vi "Field vs  IV and Ic distribution_V1.vi"() -> ()   [LabVIEW 2018]
uses:
  <vilib>/LabVIEW Targets/FPGA/cRIO/shared/nicrio_ModuleControls/nicrio_cRIO-9775_RecordDataRates4ChansRing.ctl
  <vilib>/Utility/file.llb/Write Delimited Spreadsheet (DBL).vi
  global.vi
  <resource>/objmgr/ni.dex.rc
  <vilib>/Analysis/NI_AALBase.lvlib
panel:
  in  "Tab Control":enum32{"Field", "cRIO"}(tab)
  in  "KEITHLEY 2400 GPIB Address":string="22"
  in  "Init Ramp Time s":dbl=10.0
  in  "Step Ramp Time s":dbl=1.0
  in  "Field Radius V":dbl=0.25 format="%#_13g"
  in  "Field step V":dbl=0.005 format="%#_13g"
  in  "Field Origin V":dbl format="%#_13g"
  in  "Ramp up first T":bool=TRUE
  in  "Ramp type":string(combo)="Around origin"
  in  "FIeld Scale factor":dbl=10.0
  in  "AI Channel":u8
  in  "Trigger Slope":enum8{"Positive", "Negative"}(ring)
  in  "Dist Record Samples":u32=10000
  in  "cRIO IP":string="//172.22.11.2"
  in  "Data buffer size":i32=1000
  in  "Voltage Scale factor":dbl=0.0001
  in  "Current Scale factor":dbl=2.0
  in  "IV Record Samples":u32=5000
  in  "Gate wait time us":u32=150
  in  "IV Record Data Rate":T1=200 items=["20.000 MS/s (NI 9775)"=1, "10.00 MS/s (NI 9775)"=2, "6.667 MS/s (NI 9775)"=3, "5.000 MS/s (NI 9775)"=4, "2.500 MS/s (NI 9775)"=8, "1.667 MS/s (NI 9775)"=12, "1.250 MS/s (NI 9775)"=16, "1.000 MS/s (NI 9775)"=20, "833.333 KS/s (NI 9775)"=24, "714.286 KS/s (NI 9775)"=28, "625.000 KS/s (NI 9775)"=32, "555.556 KS/s (NI 9775)"=36, "500.000 KS/s (NI 9775)"=40, "454.545 KS/s (NI 9775)"=44, "416.667 KS/s (NI 9775)"=48, "384.615 KS/s (NI 9775)"=52, "357.143 KS/s (NI 9775)"=56, "333.333 KS/s (NI 9775)"=60, "312.500 KS/s (NI 9775)"=64, "294.118 KS/s (NI 9775)"=68, "277.778 KS/s (NI 9775)"=72, "263.158 KS/s (NI 9775)"=76, "250.000 KS/s (NI 9775)"=80, "238.095 KS/s (NI 9775)"=84, "227.273 KS/s (NI 9775)"=88, "217.391 KS/s (NI 9775)"=92, "208.333 KS/s (NI 9775)"=96, "200.000 KS/s (NI 9775)"=100, "192.308 KS/s (NI 9775)"=104, "185.185 KS/s (NI 9775)"=108, "178.571 KS/s (NI 9775)"=112, "172.414 KS/s (NI 9775)"=116, "166.667 KS/s (NI 9775)"=120, "161.290 KS/s (NI 9775)"=124, "156.250 KS/s (NI 9775)"=128, "151.515 KS/s (NI 9775)"=132, "147.059 KS/s (NI 9775)"=136, "142.857 KS/s (NI 9775)"=140, "138.889 KS/s (NI 9775)"=144, "135.135 KS/s (NI 9775)"=148, "131.579 KS/s (NI 9775)"=152, "128.205 KS/s (NI 9775)"=156, "125.000 KS/s (NI 9775)"=160, "121.951 KS/s (NI 9775)"=164, "119.048 KS/s (NI 9775)"=168, "116.279 KS/s (NI 9775)"=172, "113.636 KS/s (NI 9775)"=176, "111.111 KS/s (NI 9775)"=180, "108.696 KS/s (NI 9775)"=184, "106.383 KS/s (NI 9775)"=188, "104.167 KS/s (NI 9775)"=192, "102.041 KS/s (NI 9775)"=196, "100.000 KS/s (NI 9775)"=200, "50.000 KS/s (NI 9775)"=400, "33.333 KS/s (NI 9775)"=600, "25.000 KS/s (NI 9775)"=800, "20.000 KS/s (NI 9775)"=1000, "16.667 KS/s (NI 9775)"=1200, "14.286 KS/s (NI 9775)"=1400, "12.500 KS/s (NI 9775)"=1600, "11.111 KS/s (NI 9775)"=1800, "10.000 KS/s (NI 9775)"=2000, "9.091 KS/s (NI 9775)"=2200, "8.333 KS/s (NI 9775)"=2400, "7.692 KS/s (NI 9775)"=2600, "7.143 KS/s (NI 9775)"=2800, "6.667 KS/s (NI 9775)"=3000, "6.250 KS/s (NI 9775)"=3200, "5.882 KS/s (NI 9775)"=3400, "5.556 KS/s (NI 9775)"=3600, "5.000 KS/s (NI 9775)"=4000, "4.762 KS/s (NI 9775)"=4200, "4.545 KS/s (NI 9775)"=4400, "4.348 KS/s (NI 9775)"=4600, "4.167 KS/s (NI 9775)"=4800, "4.000 KS/s (NI 9775)"=5000, "3.846 KS/s (NI 9775)"=5200, "3.571 KS/s (NI 9775)"=5600, "3.333 KS/s (NI 9775)"=6000, "3.125 KS/s (NI 9775)"=6400, "2.941 KS/s (NI 9775)"=6800, "2.778 KS/s (NI 9775)"=7200, "2.632 KS/s (NI 9775)"=7600, "2.500 KS/s (NI 9775)"=8000, "2.381 KS/s (NI 9775)"=8400, "2.273 KS/s (NI 9775)"=8800, "2.174 KS/s (NI 9775)"=9200, "2.083 KS/s (NI 9775)"=9600, "2.000 KS/s (NI 9775)"=10000, "1.923 KS/s (NI 9775)"=10400, "1.852 KS/s (NI 9775)"=10800, "1.786 KS/s (NI 9775)"=11200, "1.724 KS/s (NI 9775)"=11600, "1.667 KS/s (NI 9775)"=12000, "1.613 KS/s (NI 9775)"=12400, "1.563 KS/s (NI 9775)"=12800, "1.515 KS/s (NI 9775)"=13200, "1.471 KS/s (NI 9775)"=13600, "1.429 KS/s (NI 9775)"=14000, "1.389 KS/s (NI 9775)"=14400, "1.351 KS/s (NI 9775)"=14800, "1.316 KS/s (NI 9775)"=15200, "1.282 KS/s (NI 9775)"=15600, "1.250 KS/s (NI 9775)"=16000, "1.220 KS/s (NI 9775)"=16400, "1.190 KS/s (NI 9775)"=16800, "1.163 KS/s (NI 9775)"=17200, "1.136 KS/s (NI 9775)"=17600, "1.111 KS/s (NI 9775)"=18000, "1.087 KS/s (NI 9775)"=18400, "1.064 KS/s (NI 9775)"=18800, "1.042 KS/s (NI 9775)"=19200, "1.020 KS/s (NI 9775)"=19600, "1.000 KS/s (NI 9775)"=20000, "0.980 KS/s (NI 9775)"=20400, "0.962 KS/s (NI 9775)"=20800, "0.943 KS/s (NI 9775)"=21200, "0.926 KS/s (NI 9775)"=21600, "0.909 KS/s (NI 9775)"=22000, "0.893 KS/s (NI 9775)"=22400, "0.877 KS/s (NI 9775)"=22800, "0.862 KS/s (NI 9775)"=23200, "0.847 KS/s (NI 9775)"=23600, "0.833 KS/s (NI 9775)"=24000, "0.820 KS/s (NI 9775)"=24400, "0.806 KS/s (NI 9775)"=24800, "0.794 KS/s (NI 9775)"=25200, "0.781 KS/s (NI 9775)"=25600, "0.694 KS/s (NI 9775)"=28800, "0.625 KS/s (NI 9775)"=32000, "0.568 KS/s (NI 9775)"=35200, "0.521 KS/s (NI 9775)"=38400, "0.446 KS/s (NI 9775)"=44800, "0.391 KS/s (NI 9775)"=51200, "0.347 KS/s (NI 9775)"=57600, "0.313 KS/s (NI 9775)"=64000]
  in  "Relative threshold":dbl=0.15 format="%#_13g"
  in  "Dist Record Data Rate":T1=1 items=["20.000 MS/s (NI 9775)"=1, "10.00 MS/s (NI 9775)"=2, "6.667 MS/s (NI 9775)"=3, "5.000 MS/s (NI 9775)"=4, "2.500 MS/s (NI 9775)"=8, "1.667 MS/s (NI 9775)"=12, "1.250 MS/s (NI 9775)"=16, "1.000 MS/s (NI 9775)"=20, "833.333 KS/s (NI 9775)"=24, "714.286 KS/s (NI 9775)"=28, "625.000 KS/s (NI 9775)"=32, "555.556 KS/s (NI 9775)"=36, "500.000 KS/s (NI 9775)"=40, "454.545 KS/s (NI 9775)"=44, "416.667 KS/s (NI 9775)"=48, "384.615 KS/s (NI 9775)"=52, "357.143 KS/s (NI 9775)"=56, "333.333 KS/s (NI 9775)"=60, "312.500 KS/s (NI 9775)"=64, "294.118 KS/s (NI 9775)"=68, "277.778 KS/s (NI 9775)"=72, "263.158 KS/s (NI 9775)"=76, "250.000 KS/s (NI 9775)"=80, "238.095 KS/s (NI 9775)"=84, "227.273 KS/s (NI 9775)"=88, "217.391 KS/s (NI 9775)"=92, "208.333 KS/s (NI 9775)"=96, "200.000 KS/s (NI 9775)"=100, "192.308 KS/s (NI 9775)"=104, "185.185 KS/s (NI 9775)"=108, "178.571 KS/s (NI 9775)"=112, "172.414 KS/s (NI 9775)"=116, "166.667 KS/s (NI 9775)"=120, "161.290 KS/s (NI 9775)"=124, "156.250 KS/s (NI 9775)"=128, "151.515 KS/s (NI 9775)"=132, "147.059 KS/s (NI 9775)"=136, "142.857 KS/s (NI 9775)"=140, "138.889 KS/s (NI 9775)"=144, "135.135 KS/s (NI 9775)"=148, "131.579 KS/s (NI 9775)"=152, "128.205 KS/s (NI 9775)"=156, "125.000 KS/s (NI 9775)"=160, "121.951 KS/s (NI 9775)"=164, "119.048 KS/s (NI 9775)"=168, "116.279 KS/s (NI 9775)"=172, "113.636 KS/s (NI 9775)"=176, "111.111 KS/s (NI 9775)"=180, "108.696 KS/s (NI 9775)"=184, "106.383 KS/s (NI 9775)"=188, "104.167 KS/s (NI 9775)"=192, "102.041 KS/s (NI 9775)"=196, "100.000 KS/s (NI 9775)"=200, "50.000 KS/s (NI 9775)"=400, "33.333 KS/s (NI 9775)"=600, "25.000 KS/s (NI 9775)"=800, "20.000 KS/s (NI 9775)"=1000, "16.667 KS/s (NI 9775)"=1200, "14.286 KS/s (NI 9775)"=1400, "12.500 KS/s (NI 9775)"=1600, "11.111 KS/s (NI 9775)"=1800, "10.000 KS/s (NI 9775)"=2000, "9.091 KS/s (NI 9775)"=2200, "8.333 KS/s (NI 9775)"=2400, "7.692 KS/s (NI 9775)"=2600, "7.143 KS/s (NI 9775)"=2800, "6.667 KS/s (NI 9775)"=3000, "6.250 KS/s (NI 9775)"=3200, "5.882 KS/s (NI 9775)"=3400, "5.556 KS/s (NI 9775)"=3600, "5.000 KS/s (NI 9775)"=4000, "4.762 KS/s (NI 9775)"=4200, "4.545 KS/s (NI 9775)"=4400, "4.348 KS/s (NI 9775)"=4600, "4.167 KS/s (NI 9775)"=4800, "4.000 KS/s (NI 9775)"=5000, "3.846 KS/s (NI 9775)"=5200, "3.571 KS/s (NI 9775)"=5600, "3.333 KS/s (NI 9775)"=6000, "3.125 KS/s (NI 9775)"=6400, "2.941 KS/s (NI 9775)"=6800, "2.778 KS/s (NI 9775)"=7200, "2.632 KS/s (NI 9775)"=7600, "2.500 KS/s (NI 9775)"=8000, "2.381 KS/s (NI 9775)"=8400, "2.273 KS/s (NI 9775)"=8800, "2.174 KS/s (NI 9775)"=9200, "2.083 KS/s (NI 9775)"=9600, "2.000 KS/s (NI 9775)"=10000, "1.923 KS/s (NI 9775)"=10400, "1.852 KS/s (NI 9775)"=10800, "1.786 KS/s (NI 9775)"=11200, "1.724 KS/s (NI 9775)"=11600, "1.667 KS/s (NI 9775)"=12000, "1.613 KS/s (NI 9775)"=12400, "1.563 KS/s (NI 9775)"=12800, "1.515 KS/s (NI 9775)"=13200, "1.471 KS/s (NI 9775)"=13600, "1.429 KS/s (NI 9775)"=14000, "1.389 KS/s (NI 9775)"=14400, "1.351 KS/s (NI 9775)"=14800, "1.316 KS/s (NI 9775)"=15200, "1.282 KS/s (NI 9775)"=15600, "1.250 KS/s (NI 9775)"=16000, "1.220 KS/s (NI 9775)"=16400, "1.190 KS/s (NI 9775)"=16800, "1.163 KS/s (NI 9775)"=17200, "1.136 KS/s (NI 9775)"=17600, "1.111 KS/s (NI 9775)"=18000, "1.087 KS/s (NI 9775)"=18400, "1.064 KS/s (NI 9775)"=18800, "1.042 KS/s (NI 9775)"=19200, "1.020 KS/s (NI 9775)"=19600, "1.000 KS/s (NI 9775)"=20000, "0.980 KS/s (NI 9775)"=20400, "0.962 KS/s (NI 9775)"=20800, "0.943 KS/s (NI 9775)"=21200, "0.926 KS/s (NI 9775)"=21600, "0.909 KS/s (NI 9775)"=22000, "0.893 KS/s (NI 9775)"=22400, "0.877 KS/s (NI 9775)"=22800, "0.862 KS/s (NI 9775)"=23200, "0.847 KS/s (NI 9775)"=23600, "0.833 KS/s (NI 9775)"=24000, "0.820 KS/s (NI 9775)"=24400, "0.806 KS/s (NI 9775)"=24800, "0.794 KS/s (NI 9775)"=25200, "0.781 KS/s (NI 9775)"=25600, "0.694 KS/s (NI 9775)"=28800, "0.625 KS/s (NI 9775)"=32000, "0.568 KS/s (NI 9775)"=35200, "0.521 KS/s (NI 9775)"=38400, "0.446 KS/s (NI 9775)"=44800, "0.391 KS/s (NI 9775)"=51200, "0.347 KS/s (NI 9775)"=57600, "0.313 KS/s (NI 9775)"=64000]
  in  "Zero avg":i32=500
  out "Threshold":dbl=0.1399287109375
  in  "Stop loop":bool
  out "Current Field mT":dbl=-0.050000000000000044
  out "Current Field V":dbl=-0.0050000000000000044
  in  "Name":string="book379"
  in  "Contour plot folder":path=path "C:/Users/gyue/Box Sync/Guang Yue/data/Contour plot"
  out "Histogram Graph":T2(graph)={"X Values"=[9.09032470703125, 9.09519287109375, 9.100061035156251, 9.104929199218752, 9.109797363281253, 9.114665527343753, 9.119533691406254, 9.124401855468754, 9.129270019531255, 9.134138183593755, 9.139006347656256, 9.143874511718757, 9.148742675781257, 9.153610839843758, 9.158479003906258, 9.163347167968759, 9.16821533203126, 9.17308349609376, 9.17795166015626, 9.182819824218761, 9.187687988281262, 9.192556152343762, 9.197424316406263, 9.202292480468763, 9.207160644531264, 9.212028808593764, 9.216896972656265, 9.221765136718766, 9.226633300781266, 9.231501464843767, 9.236369628906267, 9.241237792968768, 9.246105957031268, 9.250974121093769, 9.25584228515627, 9.26071044921877, 9.26557861328127, 9.270446777343771, 9.275314941406272, 9.280183105468772, 9.285051269531273, 9.289919433593774, 9.294787597656274, 9.299655761718775, 9.304523925781275, 9.309392089843776, 9.314260253906276, 9.319128417968777, 9.323996582031278, 9.328864746093778, 9.333732910156279, 9.33860107421878, 9.34346923828128, 9.34833740234378, 9.353205566406281, 9.358073730468782, 9.362941894531282, 9.367810058593783, 9.372678222656283, 9.377546386718784, 9.382414550781284, 9.387282714843785, 9.392150878906286, 9.397019042968786, 9.401887207031287, 9.406755371093787, 9.411623535156288, 9.416491699218788, 9.421359863281289, 9.42622802734379, 9.43109619140629, 9.43596435546879, 9.440832519531291, 9.445700683593792, 9.450568847656292, 9.455437011718793, 9.460305175781293, 9.465173339843794, 9.470041503906295, 9.474909667968795, 9.479777832031296, 9.484645996093796, 9.489514160156297, 9.494382324218797, 9.499250488281298, 9.504118652343799, 9.5089868164063, 9.5138549804688, 9.5187231445313, 9.5235913085938, 9.528459472656301, 9.533327636718802, 9.538195800781303, 9.543063964843803, 9.547932128906304, 9.552800292968804, 9.557668457031305, 9.562536621093805, 9.567404785156306, 9.572272949218807], "Histogram: h(x)"=[1, 0, 0, 1, 1, 1, 0, 5, 0, 4, 3, 0, 0, 5, 6, 15, 9, 18, 14, 21, 6, 18, 23, 34, 38, 22, 54, 57, 74, 39, 98, 103, 123, 63, 111, 190, 161, 108, 207, 263, 218, 147, 272, 308, 339, 142, 370, 304, 377, 152, 388, 375, 351, 359, 135, 364, 278, 319, 146, 320, 254, 252, 130, 192, 217, 177, 103, 150, 140, 114, 62, 113, 105, 82, 24, 58, 42, 47, 16, 34, 33, 19, 18, 4, 13, 9, 7, 3, 5, 4, 2, 1, 2, 1, 2, 2, 1, 0, 0, 2]}
  out "Ic parameters":T3={"Records Num"=10000, "AI Trigger Configuration"={"Trigger Slope"=enum."Positive", "Trigger Level"=0.139892578125, "Hystesis Value"=0.1328125, "AI Channel"=0}, "Record PreTrigger Samples"=1, "Record Samples"=16, "Ic Cut off or curve"=TRUE, "Gate wait time us"=150, "Record Data Rate"=1} {"Record Data Rate" items=["20.000 MS/s (NI 9775)"=1, "10.00 MS/s (NI 9775)"=2, "6.667 MS/s (NI 9775)"=3, "5.000 MS/s (NI 9775)"=4, "2.500 MS/s (NI 9775)"=8, "1.667 MS/s (NI 9775)"=12, "1.250 MS/s (NI 9775)"=16, "1.000 MS/s (NI 9775)"=20, "833.333 KS/s (NI 9775)"=24, "714.286 KS/s (NI 9775)"=28, "625.000 KS/s (NI 9775)"=32, "555.556 KS/s (NI 9775)"=36, "500.000 KS/s (NI 9775)"=40, "454.545 KS/s (NI 9775)"=44, "416.667 KS/s (NI 9775)"=48, "384.615 KS/s (NI 9775)"=52, "357.143 KS/s (NI 9775)"=56, "333.333 KS/s (NI 9775)"=60, "312.500 KS/s (NI 9775)"=64, "294.118 KS/s (NI 9775)"=68, "277.778 KS/s (NI 9775)"=72, "263.158 KS/s (NI 9775)"=76, "250.000 KS/s (NI 9775)"=80, "238.095 KS/s (NI 9775)"=84, "227.273 KS/s (NI 9775)"=88, "217.391 KS/s (NI 9775)"=92, "208.333 KS/s (NI 9775)"=96, "200.000 KS/s (NI 9775)"=100, "192.308 KS/s (NI 9775)"=104, "185.185 KS/s (NI 9775)"=108, "178.571 KS/s (NI 9775)"=112, "172.414 KS/s (NI 9775)"=116, "166.667 KS/s (NI 9775)"=120, "161.290 KS/s (NI 9775)"=124, "156.250 KS/s (NI 9775)"=128, "151.515 KS/s (NI 9775)"=132, "147.059 KS/s (NI 9775)"=136, "142.857 KS/s (NI 9775)"=140, "138.889 KS/s (NI 9775)"=144, "135.135 KS/s (NI 9775)"=148, "131.579 KS/s (NI 9775)"=152, "128.205 KS/s (NI 9775)"=156, "125.000 KS/s (NI 9775)"=160, "121.951 KS/s (NI 9775)"=164, "119.048 KS/s (NI 9775)"=168, "116.279 KS/s (NI 9775)"=172, "113.636 KS/s (NI 9775)"=176, "111.111 KS/s (NI 9775)"=180, "108.696 KS/s (NI 9775)"=184, "106.383 KS/s (NI 9775)"=188, "104.167 KS/s (NI 9775)"=192, "102.041 KS/s (NI 9775)"=196, "100.000 KS/s (NI 9775)"=200, "50.000 KS/s (NI 9775)"=400, "33.333 KS/s (NI 9775)"=600, "25.000 KS/s (NI 9775)"=800, "20.000 KS/s (NI 9775)"=1000, "16.667 KS/s (NI 9775)"=1200, "14.286 KS/s (NI 9775)"=1400, "12.500 KS/s (NI 9775)"=1600, "11.111 KS/s (NI 9775)"=1800, "10.000 KS/s (NI 9775)"=2000, "9.091 KS/s (NI 9775)"=2200, "8.333 KS/s (NI 9775)"=2400, "7.692 KS/s (NI 9775)"=2600, "7.143 KS/s (NI 9775)"=2800, "6.667 KS/s (NI 9775)"=3000, "6.250 KS/s (NI 9775)"=3200, "5.882 KS/s (NI 9775)"=3400, "5.556 KS/s (NI 9775)"=3600, "5.000 KS/s (NI 9775)"=4000, "4.762 KS/s (NI 9775)"=4200, "4.545 KS/s (NI 9775)"=4400, "4.348 KS/s (NI 9775)"=4600, "4.167 KS/s (NI 9775)"=4800, "4.000 KS/s (NI 9775)"=5000, "3.846 KS/s (NI 9775)"=5200, "3.571 KS/s (NI 9775)"=5600, "3.333 KS/s (NI 9775)"=6000, "3.125 KS/s (NI 9775)"=6400, "2.941 KS/s (NI 9775)"=6800, "2.778 KS/s (NI 9775)"=7200, "2.632 KS/s (NI 9775)"=7600, "2.500 KS/s (NI 9775)"=8000, "2.381 KS/s (NI 9775)"=8400, "2.273 KS/s (NI 9775)"=8800, "2.174 KS/s (NI 9775)"=9200, "2.083 KS/s (NI 9775)"=9600, "2.000 KS/s (NI 9775)"=10000, "1.923 KS/s (NI 9775)"=10400, "1.852 KS/s (NI 9775)"=10800, "1.786 KS/s (NI 9775)"=11200, "1.724 KS/s (NI 9775)"=11600, "1.667 KS/s (NI 9775)"=12000, "1.613 KS/s (NI 9775)"=12400, "1.563 KS/s (NI 9775)"=12800, "1.515 KS/s (NI 9775)"=13200, "1.471 KS/s (NI 9775)"=13600, "1.429 KS/s (NI 9775)"=14000, "1.389 KS/s (NI 9775)"=14400, "1.351 KS/s (NI 9775)"=14800, "1.316 KS/s (NI 9775)"=15200, "1.282 KS/s (NI 9775)"=15600, "1.250 KS/s (NI 9775)"=16000, "1.220 KS/s (NI 9775)"=16400, "1.190 KS/s (NI 9775)"=16800, "1.163 KS/s (NI 9775)"=17200, "1.136 KS/s (NI 9775)"=17600, "1.111 KS/s (NI 9775)"=18000, "1.087 KS/s (NI 9775)"=18400, "1.064 KS/s (NI 9775)"=18800, "1.042 KS/s (NI 9775)"=19200, "1.020 KS/s (NI 9775)"=19600, "1.000 KS/s (NI 9775)"=20000, "0.980 KS/s (NI 9775)"=20400, "0.962 KS/s (NI 9775)"=20800, "0.943 KS/s (NI 9775)"=21200, "0.926 KS/s (NI 9775)"=21600, "0.909 KS/s (NI 9775)"=22000, "0.893 KS/s (NI 9775)"=22400, "0.877 KS/s (NI 9775)"=22800, "0.862 KS/s (NI 9775)"=23200, "0.847 KS/s (NI 9775)"=23600, "0.833 KS/s (NI 9775)"=24000, "0.820 KS/s (NI 9775)"=24400, "0.806 KS/s (NI 9775)"=24800, "0.794 KS/s (NI 9775)"=25200, "0.781 KS/s (NI 9775)"=25600, "0.694 KS/s (NI 9775)"=28800, "0.625 KS/s (NI 9775)"=32000, "0.568 KS/s (NI 9775)"=35200, "0.521 KS/s (NI 9775)"=38400, "0.446 KS/s (NI 9775)"=44800, "0.391 KS/s (NI 9775)"=51200, "0.347 KS/s (NI 9775)"=57600, "0.313 KS/s (NI 9775)"=64000]}
  out "IV parameters":T3={"Records Num"=1, "AI Trigger Configuration"={"Trigger Slope"=enum."Positive", "Trigger Level"=0.10009765625, "Hystesis Value"=0.094970703125, "AI Channel"=0}, "Record PreTrigger Samples"=1, "Record Samples"=5000, "Ic Cut off or curve"=FALSE, "Gate wait time us"=150, "Record Data Rate"=200} {"Record Data Rate" items=["20.000 MS/s (NI 9775)"=1, "10.00 MS/s (NI 9775)"=2, "6.667 MS/s (NI 9775)"=3, "5.000 MS/s (NI 9775)"=4, "2.500 MS/s (NI 9775)"=8, "1.667 MS/s (NI 9775)"=12, "1.250 MS/s (NI 9775)"=16, "1.000 MS/s (NI 9775)"=20, "833.333 KS/s (NI 9775)"=24, "714.286 KS/s (NI 9775)"=28, "625.000 KS/s (NI 9775)"=32, "555.556 KS/s (NI 9775)"=36, "500.000 KS/s (NI 9775)"=40, "454.545 KS/s (NI 9775)"=44, "416.667 KS/s (NI 9775)"=48, "384.615 KS/s (NI 9775)"=52, "357.143 KS/s (NI 9775)"=56, "333.333 KS/s (NI 9775)"=60, "312.500 KS/s (NI 9775)"=64, "294.118 KS/s (NI 9775)"=68, "277.778 KS/s (NI 9775)"=72, "263.158 KS/s (NI 9775)"=76, "250.000 KS/s (NI 9775)"=80, "238.095 KS/s (NI 9775)"=84, "227.273 KS/s (NI 9775)"=88, "217.391 KS/s (NI 9775)"=92, "208.333 KS/s (NI 9775)"=96, "200.000 KS/s (NI 9775)"=100, "192.308 KS/s (NI 9775)"=104, "185.185 KS/s (NI 9775)"=108, "178.571 KS/s (NI 9775)"=112, "172.414 KS/s (NI 9775)"=116, "166.667 KS/s (NI 9775)"=120, "161.290 KS/s (NI 9775)"=124, "156.250 KS/s (NI 9775)"=128, "151.515 KS/s (NI 9775)"=132, "147.059 KS/s (NI 9775)"=136, "142.857 KS/s (NI 9775)"=140, "138.889 KS/s (NI 9775)"=144, "135.135 KS/s (NI 9775)"=148, "131.579 KS/s (NI 9775)"=152, "128.205 KS/s (NI 9775)"=156, "125.000 KS/s (NI 9775)"=160, "121.951 KS/s (NI 9775)"=164, "119.048 KS/s (NI 9775)"=168, "116.279 KS/s (NI 9775)"=172, "113.636 KS/s (NI 9775)"=176, "111.111 KS/s (NI 9775)"=180, "108.696 KS/s (NI 9775)"=184, "106.383 KS/s (NI 9775)"=188, "104.167 KS/s (NI 9775)"=192, "102.041 KS/s (NI 9775)"=196, "100.000 KS/s (NI 9775)"=200, "50.000 KS/s (NI 9775)"=400, "33.333 KS/s (NI 9775)"=600, "25.000 KS/s (NI 9775)"=800, "20.000 KS/s (NI 9775)"=1000, "16.667 KS/s (NI 9775)"=1200, "14.286 KS/s (NI 9775)"=1400, "12.500 KS/s (NI 9775)"=1600, "11.111 KS/s (NI 9775)"=1800, "10.000 KS/s (NI 9775)"=2000, "9.091 KS/s (NI 9775)"=2200, "8.333 KS/s (NI 9775)"=2400, "7.692 KS/s (NI 9775)"=2600, "7.143 KS/s (NI 9775)"=2800, "6.667 KS/s (NI 9775)"=3000, "6.250 KS/s (NI 9775)"=3200, "5.882 KS/s (NI 9775)"=3400, "5.556 KS/s (NI 9775)"=3600, "5.000 KS/s (NI 9775)"=4000, "4.762 KS/s (NI 9775)"=4200, "4.545 KS/s (NI 9775)"=4400, "4.348 KS/s (NI 9775)"=4600, "4.167 KS/s (NI 9775)"=4800, "4.000 KS/s (NI 9775)"=5000, "3.846 KS/s (NI 9775)"=5200, "3.571 KS/s (NI 9775)"=5600, "3.333 KS/s (NI 9775)"=6000, "3.125 KS/s (NI 9775)"=6400, "2.941 KS/s (NI 9775)"=6800, "2.778 KS/s (NI 9775)"=7200, "2.632 KS/s (NI 9775)"=7600, "2.500 KS/s (NI 9775)"=8000, "2.381 KS/s (NI 9775)"=8400, "2.273 KS/s (NI 9775)"=8800, "2.174 KS/s (NI 9775)"=9200, "2.083 KS/s (NI 9775)"=9600, "2.000 KS/s (NI 9775)"=10000, "1.923 KS/s (NI 9775)"=10400, "1.852 KS/s (NI 9775)"=10800, "1.786 KS/s (NI 9775)"=11200, "1.724 KS/s (NI 9775)"=11600, "1.667 KS/s (NI 9775)"=12000, "1.613 KS/s (NI 9775)"=12400, "1.563 KS/s (NI 9775)"=12800, "1.515 KS/s (NI 9775)"=13200, "1.471 KS/s (NI 9775)"=13600, "1.429 KS/s (NI 9775)"=14000, "1.389 KS/s (NI 9775)"=14400, "1.351 KS/s (NI 9775)"=14800, "1.316 KS/s (NI 9775)"=15200, "1.282 KS/s (NI 9775)"=15600, "1.250 KS/s (NI 9775)"=16000, "1.220 KS/s (NI 9775)"=16400, "1.190 KS/s (NI 9775)"=16800, "1.163 KS/s (NI 9775)"=17200, "1.136 KS/s (NI 9775)"=17600, "1.111 KS/s (NI 9775)"=18000, "1.087 KS/s (NI 9775)"=18400, "1.064 KS/s (NI 9775)"=18800, "1.042 KS/s (NI 9775)"=19200, "1.020 KS/s (NI 9775)"=19600, "1.000 KS/s (NI 9775)"=20000, "0.980 KS/s (NI 9775)"=20400, "0.962 KS/s (NI 9775)"=20800, "0.943 KS/s (NI 9775)"=21200, "0.926 KS/s (NI 9775)"=21600, "0.909 KS/s (NI 9775)"=22000, "0.893 KS/s (NI 9775)"=22400, "0.877 KS/s (NI 9775)"=22800, "0.862 KS/s (NI 9775)"=23200, "0.847 KS/s (NI 9775)"=23600, "0.833 KS/s (NI 9775)"=24000, "0.820 KS/s (NI 9775)"=24400, "0.806 KS/s (NI 9775)"=24800, "0.794 KS/s (NI 9775)"=25200, "0.781 KS/s (NI 9775)"=25600, "0.694 KS/s (NI 9775)"=28800, "0.625 KS/s (NI 9775)"=32000, "0.568 KS/s (NI 9775)"=35200, "0.521 KS/s (NI 9775)"=38400, "0.446 KS/s (NI 9775)"=44800, "0.391 KS/s (NI 9775)"=51200, "0.347 KS/s (NI 9775)"=57600, "0.313 KS/s (NI 9775)"=64000]}
  out "XY Graph":cluster{"Y":dbl[], "Y":dbl[]}[](graph)
  in  "stop":bool
  out "error out":errorcluster={"status"=FALSE, "code"=180121605, "source"="Shared Variable in Field vs  IV and Ic distribution.vi<APPEND>\nThis error or warning occurred while writing the following Shared Variable:\n\\\\NI-cRIO-9063-01bc8cc6\\network varibles\\RT Stop\n\\\\172.22.11.2\\network varibles\\RT Stop"}
  # "Voltage x factor=mT"
  # "Distribution setting"
  # "IV setting"
  # "Voltage x factor=uA"
  # "Voltage x factor=V"
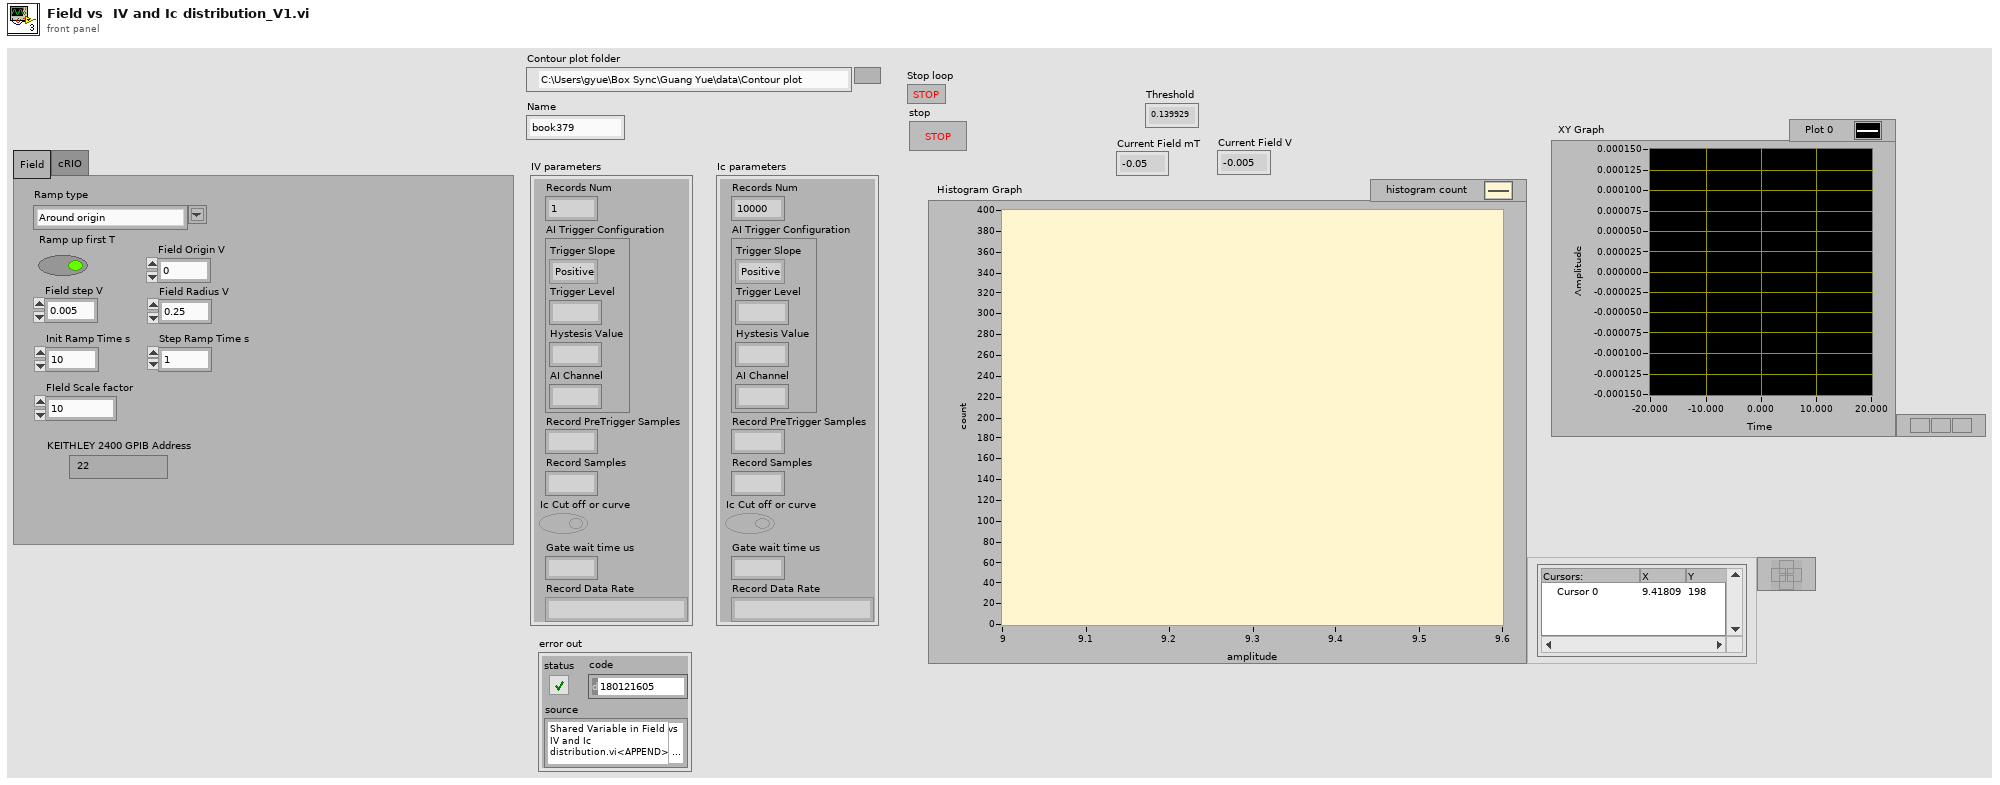
[diagram p1: front panel]
types:
  T1 = typedef "nicrio_cRIO-9775_RecordDataRates4ChansRing.ctl" = u16
  T2 = cluster{"X Values":dbl[], "Histogram: h(x)":i32[]}
  T3 = cluster{"Records Num":i32, "AI Trigger Configuration":cluster{"Trigger Slope":enum8{"Positive", "Negative"}, "Trigger Level":fxp<+/-,17,5>, "Hystesis Value":fxp<+,16,4>, "AI Channel":u8}, "Record PreTrigger Samples":u32, "Record Samples":u32, "Ic Cut off or curve":bool, "Gate wait time us":u32, "Record Data Rate":T1}
  T4 = cluster{"Trigger Slope":enum8{"Positive", "Negative"}, "Trigger Level":fxp<+/-,17,5>, "Hystesis Value":fxp<+,16,4>, "AI Channel":u8}
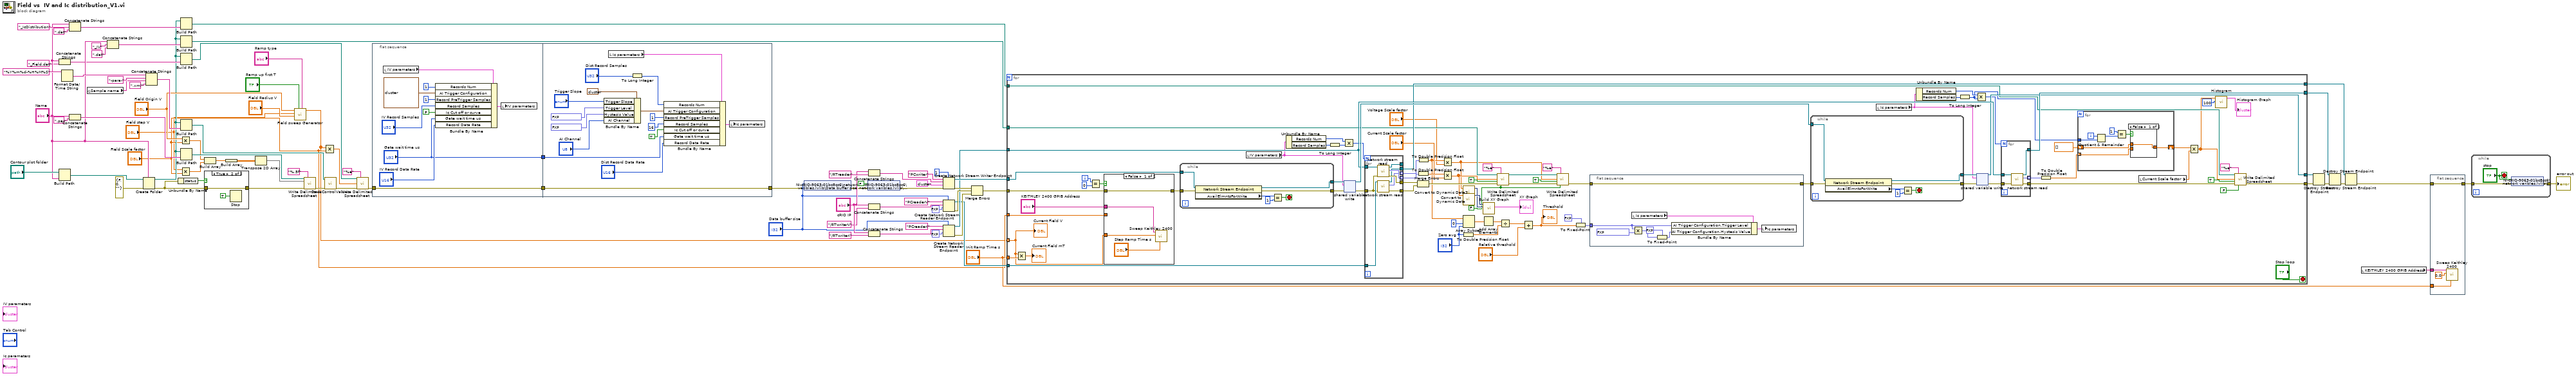
[diagram p0: block diagram]
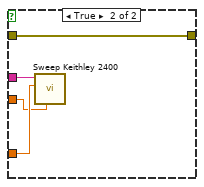
[diagram p3: hidden frame]
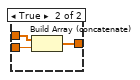
[diagram p4: hidden frame]
diagram:
  n1 = Concatenate Strings("Name", "_Field.dat" ("string")) -> (w14:string)
  n2 = Build Path(base path="Contour plot folder", name or relative path="Name") -> (appended path=w40:path)
  n3 = Format Date/Time String(time format string (%c)="%Y%m%d-%H%M%S") -> (date/time string=w35:string)  [unwired: 2 in]
  n4 = Concatenate Strings("Name", "_IcDistribution" ("string"), ".dat" ("string")) -> (w26:string)
  n5 = Concatenate Strings("Name", ".par" ("string")) -> (w47:string)
  n6 = global read "global.vi" "Sample name"() -> (w34:string)
  n7 = Concatenate Strings("Name", "_IV" ("string"), ".dat" ("string")) -> (w41:string)
  n8 = Create Folder(prompt (Create Folder)="Name", path (use dialog)=w40, error in=errorcluster {"status"=FALSE, "code"=0, "source"=""}) -> (created path=w13:path, error out=w37:errorcluster)  [unwired: 1 out]
  n9 = Concatenate Strings(w35, "-para-" ("string"), w34, ".xml" ("string")) -> (w51:string)
  n10 = Unbundle By Name(w37) -> ("status"=w38:bool)
  n11 = Multiply(x="Field Origin V", y="FIeld Scale factor") -> (x*y=w33:dbl)
  n12 = Multiply(x="Field step V", y="FIeld Scale factor") -> (x*y=w32:dbl)
  n13 = Build Path(base path=w13, name or relative path=w26) -> (appended path=w24:path)
  n14 = Build Path(base path=w13, name or relative path=w41) -> (appended path=w25:path)
  n15 = Build Path(base path=w13, name or relative path=w14) -> (appended path=w12:path)
  n16 = Build Path(base path=w13, name or relative path=w51) -> (appended path=w49:path)
  n17 = Build Path(base path=w13, name or relative path=w47) -> (appended path=w46:path)
  n18 = Build Array(w33, w32) -> (w44:dbl[])
  n19 = case shown="True" w38 {
    tunnel: [w87 w89] -> w36
    tunnel: w37 -> [w87 w89]
    frame False {
    }
    frame True {
      n20 = Stop(stop? (T)=TRUE) -> ()
    }
  }
  n21 = Build Array(w44) -> (w43:dbl[][])
  n22 = Transpose 2D Array(2D array=w43) -> (transposed array=w42:dbl[][])
  n23 = call "Field sweep Generator.vi"("Ramp type"="Ramp type", "Ramp up first T"="Ramp up first T", "Field Radius V"="Field Radius V", "Field step V"="Field step V", "Field Origin V"="Field Origin V") -> ("output array"=w3:dbl[])  [unwired: 6 in]
  n24 = call-poly <vilib>:"Write Delimited Spreadsheet.vi"("file path (dialog if empty)"=w46, "format (%.3f)"="%.5f", "2D data"=w42, "error in (no error)"=w36) -> ("error out"=w39:errorcluster)  [unwired: 10 in, 1 out]
  n25 = Multiply(x=w3, y="FIeld Scale factor") -> (x*y=w9:dbl[])
  n26 = call "SaveControlValues.vi"("XML File Path"=w49, "error in (no error)"=w39) -> ("error out"=w8:errorcluster)  [unwired: 8 in]
  n27 = call-poly <vilib>:"Write Delimited Spreadsheet.vi"("file path (dialog if empty)"=w12, "format (%.3f)"="%e", "1D data"=w9, "error in (no error)"=w8) -> ("error out"=w7:errorcluster)  [unwired: 10 in, 1 out]
  n28 = flat-sequence {
    tunnel: w7 -> [w99]
    tunnel: [w99] -> w5
    tunnel: ["Gate wait time us"] -> w4
    tunnel: [w115] -> w6
    tunnel: w5 -> [w115]
    tunnel: w4 -> [w107]
    frame #0 {
      n29 = local read "IV parameters"() -> (w98:T3)
      n30 = Bundle By Name(cluster=w98, "Records Num"=1, "AI Trigger Configuration"=T4 {"Trigger Slope"=enum."Positive", "Trigger Level"=0.10009765625, "Hystesis Value"=0.094970703125, "AI Channel"=0}, "Record PreTrigger Samples"=u32 1, "Record Samples"="IV Record Samples", "Ic Cut off or curve"=FALSE, "Gate wait time us"="Gate wait time us", "Record Data Rate"="IV Record Data Rate") -> (w90:T3)
      n31 = local write "IV parameters"(w90) -> ()
    }
    frame #1 {
      n32 = Bundle By Name(cluster=T4 {"Trigger Slope"=enum."Positive", "Trigger Level"=0.1708984375, "Hystesis Value"=0.162353515625, "AI Channel"=0} ("AI Trigger Configuration"), "Trigger Slope"="Trigger Slope", "Trigger Level"=fxp<+/-,17,5> 0.14990234375, "Hystesis Value"=fxp<+,16,4> 0.10009765625, "AI Channel"="AI Channel") -> (w103:T4)
      n33 = local read "Ic parameters"() -> (w114:T3)
      n34 = To Long Integer(number="Dist Record Samples") -> (32bit integer=w112:i32)
      n35 = Bundle By Name(cluster=w114, "Records Num"=w112, "AI Trigger Configuration"=w103, "Record PreTrigger Samples"=u32 1, "Record Samples"=u32 16, "Ic Cut off or curve"=TRUE, "Gate wait time us"=w107, "Record Data Rate"="Dist Record Data Rate") -> (w102:T3)
      n36 = local write "Ic parameters"(w102) -> ()
    }
  }
  n37 = shared-variable "NI-cRIO-9063-01bc8cc6\\network varibles.lvlib\\Data buffer size"("Data buffer size", error in=w6) -> (error out=w64:errorcluster)
  n38 = shared-variable "NI-cRIO-9063-01bc8cc6\\network varibles.lvlib\\RT Stop"(FALSE ("RT Stop"), error in=w64) -> (error out=w72:errorcluster)
  n39 = Concatenate Strings("cRIO IP", "/RTreader" ("string")) -> (w82:string)
  n40 = Concatenate Strings("cRIO IP", "/RTwriterV" ("string")) -> (w74:string)
  n41 = Concatenate Strings("cRIO IP", "/RTwriterI" ("string")) -> (w66:string)
  n42 = Create Network Stream Writer Endpoint(7:1 ("writer buffer size"), 8:w72, 9:T3 {"Records Num"=0, "AI Trigger Configuration"={"Trigger Slope"=enum."Positive", "Trigger Level"=0.0, "Hystesis Value"=0.0, "AI Channel"=0}, "Record PreTrigger Samples"=0, "Record Samples"=0, "Ic Cut off or curve"=FALSE, "Gate wait time us"=0, "Record Data Rate"=1} ("Parameters 4"), 10:w82, 11:"PCwriter" ("writer name")) -> (0:w80:errorcluster, 3:w79:refnum<k21>)  [unwired: 2 in]
  n43 = Create Network Stream Reader Endpoint(7:"Data buffer size", 9:fxp<+/-,17,5> 0.0, 10:w74, 11:"PCreaderV" ("reader name")) -> (0:w71:errorcluster, 3:w58:refnum<k21>)  [unwired: 3 in]
  n44 = Create Network Stream Reader Endpoint(7:"Data buffer size", 9:fxp<+/-,17,5> 0.0, 10:w66, 11:"PCreaderI" ("reader name")) -> (0:w63:errorcluster, 3:w61:refnum<k21>)  [unwired: 3 in]
  n45 = Merge Errors(w80, w71, w63) -> (w78:errorcluster)
  n46 = for {
    tunnel: w79 -> [w196]
    tunnel: [w185] -> w59
    tunnel: w78 -> [w158]
    tunnel: [w143] -> w56
    tunnel: w61 -> [w190]
    tunnel: [w188] -> w60
    tunnel: w58 -> [w173]
    tunnel: [w172] -> w57
    tunnel: "FIeld Scale factor" -> [w162]
    tunnel: "Init Ramp Time s" -> [w159]
    tunnel: w25 -> [w149]
    tunnel: w24 -> [w141]
    tunnel: w3 -> [w126] mode=indexing
    i -> [w163]
    stop <- "Stop loop" stop-if-true
    w127 = FALSE ("transpose? (no:F)")
    n47 = Multiply(x=w126, y=w162) -> (x*y=→"Current Field mT":dbl)
    n48 = Equal?(x=w163, y=0) -> (x = y?=w161:bool)
    n49 = case shown="False" w161 {
      tunnel: w158 -> [w209 w210]
      tunnel: [w209 w210] -> w157
      tunnel: w126 -> [w206 w213]
      tunnel: "KEITHLEY 2400 GPIB Address" -> [w207 w212]
      tunnel: w159 -> [_ w211]
      frame False {
        n50 = call "Sweep Keithley 2400.vi"("Ramp Time (s)"="Step Ramp Time s", "final gate voltage (V)"=w206, "KEITHLEY 2400 GPIB Address"=w207) -> ()  [unwired: 7 in, 2 out]
      }
      frame True {
        n51 = call "Sweep Keithley 2400.vi"("Ramp Time (s)"=w211, "final gate voltage (V)"=w213, "KEITHLEY 2400 GPIB Address"=w212) -> ()  [unwired: 7 in, 2 out]
      }
    }
    n52 = while {
      tunnel: w196 -> [w253]
      tunnel: w157 -> [w252]
      tunnel: [w248] -> w197
      tunnel: [w247] -> w195
      stop <- w249 stop-if-true
      n53 = property class="Network Stream Endpoint"(reference=w253, error in=w252) -> (reference out=w248:refnum<k21>, error out=w247:errorcluster, "AvailElmntsForWrite"=w251:i32)
      n54 = Equal?(x=w251, y=1) -> (x = y?=w249:bool)
    }
    n55 = local read "IV parameters"() -> (w178:T3)
    n56 = Unbundle By Name(w178) -> ("Records Num"=w177:i32, "Record Samples"=w176:u32)
    n57 = To Long Integer(number=w176) -> (32bit integer=w175:i32)
    n58 = Multiply(x=w177, y=w175) -> (x*y=w174:i32)
    n59 = shared-variable-write(w197, w195, w178) -> (w193:refnum<k21>, w194:errorcluster)  [unwired: 1 in, 1 out]
    n60 = for {
      N: w174 -> [_]
      tunnel: w190 -> [w246]
      tunnel: w194 -> [w239]
      tunnel: [w245] -> w148 mode=indexing
      tunnel: [w244] -> _
      tunnel: [w243] -> w171
      tunnel: w173 -> [w242]
      tunnel: [w241] -> w172
      tunnel: [w240] -> w147 mode=indexing
      tunnel: [w238] -> w170
      n61 = call "network stream read.vi"("error in (no error)"=w239, "endpoint in"=w246) -> ("error out"=w243:errorcluster, "Data"=w245:fxp<+/-,17,5>, "endpoint out"=w244:refnum<k21>)  [unwired: 7 in]
      n62 = call "network stream read.vi"("error in (no error)"=w239, "endpoint in"=w242) -> ("error out"=w238:errorcluster, "Data"=w240:fxp<+/-,17,5>, "endpoint out"=w241:refnum<k21>)  [unwired: 7 in]
    }
    n63 = To Double Precision Float(number=w148) -> (double precision float=w125:dbl[])
    n64 = Merge Errors(w171, w170) -> (w154:errorcluster)
    n65 = To Double Precision Float(number=w147) -> (double precision float=w122:dbl[])
    n66 = Multiply(x=w122, y="Voltage Scale factor") -> (x*y=w120:dbl[])
    n67 = Multiply(x=w125, y="Current Scale factor") -> (x*y=w123:dbl[])
    n68 = call "Convert to Dynamic Data2"("Array"=w120) -> ("Dynamic Data Type"=w183:dynamicdata)  [unwired: 3 in]
    n69 = call "Convert to Dynamic Data"("Array"=w123) -> ("Dynamic Data Type"=w184:dynamicdata)  [unwired: 3 in]
    n70 = Array Subset(array=w122, index=0, length="Zero avg") -> (w138:dbl[])
    n71 = To Double Precision Float(number="Zero avg") -> (double precision float=w135:dbl)
    n72 = Add Array Elements(numeric array=w138) -> (sum=w137:dbl)
    n73 = call "Build XY Graph"("Y Input"=w183, "X Input"=w184) -> ("XY Graph"=→"XY Graph":cluster{"X":dbl[], "Y":dbl[]}[])  [unwired: 8 in, 1 out]
    n74 = call-poly <vilib>:"Write Delimited Spreadsheet.vi"("file path (dialog if empty)"=w149, "format (%.3f)"="%e", "1D data"=w123, "append to file? (new file:F)"=TRUE, "error in (no error)"=w154, "transpose? (no:F)"=w127) -> ("new file path (Not A Path if cancelled)"=w150:path, "error out"=w151:errorcluster)  [unwired: 8 in]
    n75 = Divide(x=w137, y=w135) -> (x/y=w134:dbl)
    n76 = Add(x=w134, y="Relative threshold") -> (x+y=w116:dbl)
    "Threshold" <- w116
    n77 = call-poly <vilib>:"Write Delimited Spreadsheet.vi"("file path (dialog if empty)"=w150, "format (%.3f)"="%e", "1D data"=w120, "append to file? (new file:F)"=TRUE, "error in (no error)"=w151, "transpose? (no:F)"=w127) -> ("error out"=w130:errorcluster)  [unwired: 8 in, 1 out]
    n78 = To Fixed-Point(fixed-point type=fxp<+,16,4> 0.0 ("AI Trigger Configuration.Hystesis Value"), number=w116) -> (fixed-point=w132:fxp<+,16,4>)
    n79 = flat-sequence {
      tunnel: w132 -> [w202]
      tunnel: w130 -> [w203]
      tunnel: [w203] -> w129
      frame #0 {
        n80 = local read "Ic parameters"() -> (w205:T3)
        n81 = Multiply(x=w202, y=fxp<+,16,4> 0.949951171875) -> (x*y=w199:fxp<+,32,8>)
        n82 = To Fixed-Point(fixed-point type=fxp<+,16,4> 0.0 ("AI Trigger Configuration.Hystesis Value"), number=w199) -> (fixed-point=w200:fxp<+,16,4>)
        n83 = Bundle By Name(cluster=w205, "AI Trigger Configuration.Trigger Level"=w202, "AI Trigger Configuration.Hystesis Value"=w200) -> (w204:T3)
        n84 = local write "Ic parameters"(w204) -> ()
      }
    }
    n85 = while {
      tunnel: w193 -> [w235]
      tunnel: w129 -> [w234]
      tunnel: [w232] -> w192
      tunnel: [w231] -> w191
      stop <- w233 stop-if-true
      n86 = property class="Network Stream Endpoint"(reference=w235, error in=w234) -> (reference out=w232:refnum<k21>, error out=w231:errorcluster, "AvailElmntsForWrite"=w237:i32)
      n87 = Equal?(x=w237, y=1) -> (x = y?=w233:bool)
    }
    n88 = local read "Ic parameters"() -> (w182:T3)
    n89 = Unbundle By Name(w182) -> ("Records Num"=w181:i32, "Record Samples"=w180:u32)
    n90 = To Long Integer(number=w180) -> (32bit integer=w167:i32)
    n91 = Multiply(x=w181, y=w167) -> (x*y=w179:i32)
    n92 = shared-variable-write(w192, w191, w182) -> (w185:refnum<k21>, w189:errorcluster)  [unwired: 1 in, 1 out]
    n93 = for {
      N: w179 -> [_]
      tunnel: w190 -> [w230]
      tunnel: w189 -> [w229]
      tunnel: [w228] -> w144
      tunnel: [w227] -> w188
      tunnel: [w226] -> w186 mode=indexing
      n94 = call "network stream read.vi"("error in (no error)"=w229, "endpoint in"=w230) -> ("error out"=w228:errorcluster, "Data"=w226:fxp<+/-,17,5>, "endpoint out"=w227:refnum<k21>)  [unwired: 7 in]
    }
    n95 = To Double Precision Float(number=w186) -> (double precision float=w142:dbl[])
    n96 = for {
      tunnel: w142 -> [w215] mode=indexing
      tunnel: w167 -> [w221]
      shift-right: [w217] -> w119
      shift-left: dbl[] [] -> [w216]
      i -> [w220]
      n97 = Quotient & Remainder(x=w220, y=w221) -> (x-y*floor(x/y)=w219:i32)  [unwired: 1 out]
      n98 = Equal?(x=1, y=w219) -> (x = y?=w214:bool)
      n99 = case shown="False" w214 {
        tunnel: [w222 w225] -> w217
        tunnel: w216 -> [w222 w224]
        tunnel: w215 -> [_ w223]
        frame False {
        }
        frame True {
          n100 = Build Array (concatenate)(w224, w223) -> (w225:dbl[])
        }
      }
    }
    n101 = local read "Current Scale factor"() -> (w117:dbl)
    n102 = Multiply(x=w119, y=w117) -> (x*y=w118:dbl[])
    n103 = call <vilib>:"Histogram.vi"("intervals"=100, "X"=w118) -> ("Histogram Graph"=→"Histogram Graph":T2)  [unwired: 6 in, 3 out]
    n104 = call-poly <vilib>:"Write Delimited Spreadsheet.vi"("file path (dialog if empty)"=w141, "format (%.3f)"="%e", "1D data"=w118, "append to file? (new file:F)"=TRUE, "error in (no error)"=w144, "transpose? (no:F)"=FALSE) -> ("error out"=w143:errorcluster)  [unwired: 8 in, 1 out]
    "Current Field V" <- w126
  }
  n105 = Destroy Stream Endpoint(8:w56, 11:w59) -> (0:w70:errorcluster)
  n106 = Destroy Stream Endpoint(8:w70, 11:w60) -> (0:w62:errorcluster)
  n107 = Destroy Stream Endpoint(8:w62, 11:w57) -> (0:w20:errorcluster)
  n108 = local read "KEITHLEY 2400 GPIB Address"() -> (w21:string)
  n109 = flat-sequence {
    tunnel: w20 -> [w257]
    tunnel: [w257] -> w23
    tunnel: "Init Ramp Time s" -> [w256]
    tunnel: w21 -> [w254]
    frame #0 {
      n110 = call "Sweep Keithley 2400.vi"("Ramp Time (s)"=w256, "final gate voltage (V)"=0.0, "KEITHLEY 2400 GPIB Address"=w254) -> ()  [unwired: 7 in, 2 out]
    }
  }
  n111 = while {
    tunnel: w23 -> [w259]
    tunnel: [w258] -> w69
    stop <- "stop" stop-if-true
    n112 = shared-variable "NI-cRIO-9063-01bc8cc6\\network varibles.lvlib\\RT Stop"("stop", error in=w259) -> (error out=w258:errorcluster)
  }
  "error out" <- w69
